vi "Write Temperature to Logfile.vi"(0 "tdms file":refnum<k34>, 5 "Tube Temperature (K)":dbl, 7 "Manifold Temperature (K)":dbl, 9 "Ambient Temperature (K)":dbl, 11 "error in (no error)":errorcluster) -> (4 "tdms file out":refnum<k34>, 15 "error out":errorcluster)   [LabVIEW 2018]
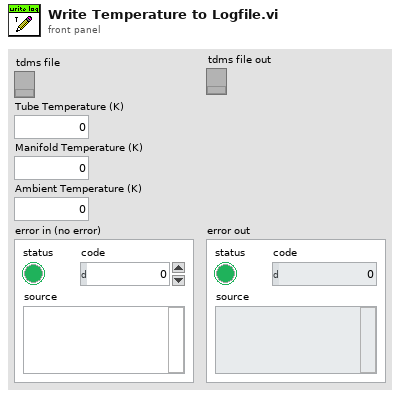
[diagram p1: front panel]
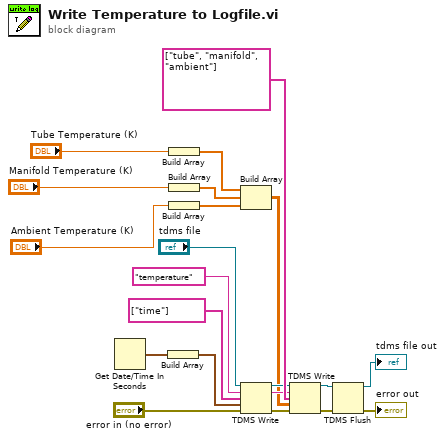
[diagram p0: block diagram]
diagram:
  n1 = Get Date/Time In Seconds() -> (seconds since 1Jan1904=w17:timestamp)
  n2 = Build Array(w17) -> (w16:timestamp[])
  n3 = Build Array("Tube Temperature (K)") -> (w11:dbl[])
  n4 = Build Array("Manifold Temperature (K)") -> (w10:dbl[])
  n5 = Build Array("Ambient Temperature (K)") -> (w2:dbl[])
  n6 = Build Array(w11, w10, w2) -> (w9:dbl[][])
  n7 = TDMS Write(0:"tdms file", 5:"temperature" ("group name in (Untitled)"), 7:string[] ["time"] ("channel name(s) in (Untitled)"), 9:w16, 11:"error in (no error)") -> (4:w15:refnum<k34>, 6:w14:string, 15:w18:errorcluster)  [unwired: 1 in, 1 out]
  n8 = TDMS Write(0:w15, 5:w14, 7:string[] ["tube", "manifold", "ambient"] ("channel name(s) in (Untitled)"), 9:w9, 11:w18) -> (4:w20:refnum<k34>, 15:w21:errorcluster)  [unwired: 1 in, 2 out]
  n9 = TDMS Flush(4:w21, 7:w20) -> (0:→"error out":errorcluster, 3:→"tdms file out":refnum<k34>)
